vi "Log Part Ttype.vi"(8 "error in (no error)":errorcluster caption="错误输入（无错误）", 11 "Base":path) -> (0 "error out":errorcluster, 3 "添加的路径":path)   [LabVIEW 2014]
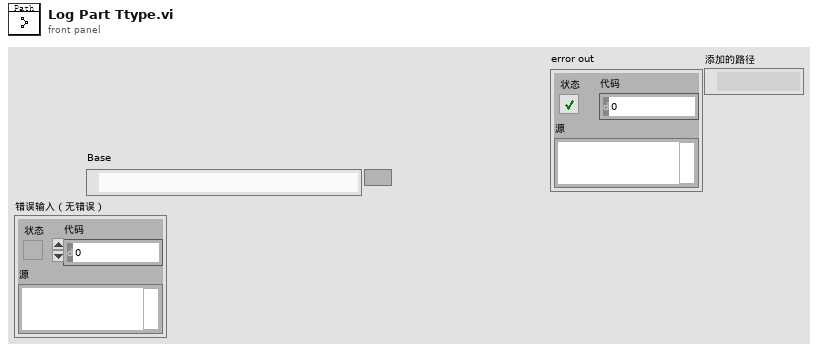
[diagram p1: front panel]
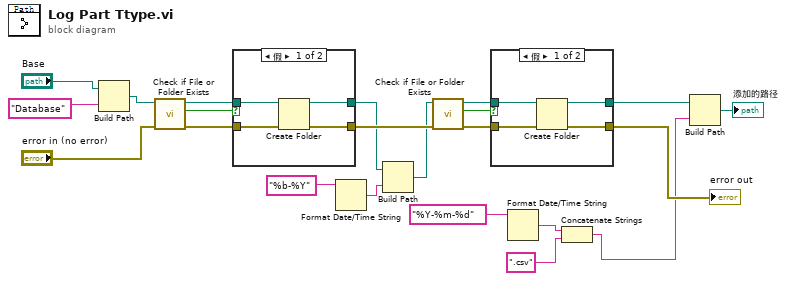
[diagram p0: block diagram]
diagram:
  n1 = Build Path(base path="Base", name or relative path="Database") -> (appended path=w2:path)
  n2 = call <vilib>:"Check if File or Folder Exists.vi"("error in (no error)"="error in (no error)", "path"=w2) -> ("error out"=w20:errorcluster, "file or folder exists?"=w21:bool, "dup path"=w19:path)  [unwired: 7 in]
  n3 = case shown="假" w21 {
    tunnel: w20 -> [w26 w27]
    tunnel: w19 -> [w25 w28]
    tunnel: [w24 w28] -> w13
    tunnel: [w23 w27] -> w15
    frame False {
      n4 = Create Folder(path (use dialog)=w25, error in=w26) -> (created path=w24:path, error out=w23:errorcluster)  [unwired: 1 in, 1 out]
    }
    frame True {
    }
  }
  n5 = Format Date/Time String(time format string (%c)="%b-%Y") -> (date/time string=w11:string)  [unwired: 2 in]
  n6 = Build Path(base path=w13, name or relative path=w11) -> (appended path=w14:path)
  n7 = call <vilib>:"Check if File or Folder Exists.vi"("error in (no error)"=w15, "path"=w14) -> ("error out"=w17:errorcluster, "file or folder exists?"=w18:bool, "dup path"=w16:path)  [unwired: 7 in]
  n8 = case shown="假" w18 {
    tunnel: w17 -> [w32 w33]
    tunnel: w16 -> [w31 w34]
    tunnel: [w30 w34] -> w10
    tunnel: [w29 w33] -> w9
    frame False {
      n9 = Create Folder(path (use dialog)=w31, error in=w32) -> (created path=w30:path, error out=w29:errorcluster)  [unwired: 1 in, 1 out]
    }
    frame True {
    }
  }
  "error out" <- w9
  n10 = Format Date/Time String(time format string (%c)="%Y-%m-%d") -> (date/time string=w6:string)  [unwired: 2 in]
  n11 = Concatenate Strings(w6, ".csv") -> (w4:string)
  n12 = Build Path(base path=w10, name or relative path=w4) -> (appended path=→"添加的路径":path)
